vi "Proc_ccdIV.vi"(11 "error in (no error)":errorcluster, 12 "logfile":path, 13 "Database RefNum out":T1) -> (15 "error out":errorcluster)   [LabVIEW 2016]
uses:
  DBSHAND/private/vis/DatabaseHand_RefNum.ctl
  Common/public/vis/CMN_FVAR_action.ctl
  DBSHAND/private/vis/DatabaseHand_Element_Get(double).vi
  DBSHAND/private/vis/DatabaseHand_Element_Set(double).vi
  DBSHAND/private/vis/DatabaseHand_Element_Set(bool).vi
  DBSHAND/private/vis/DatabaseHand_Element_Get(I32).vi
  DBSHAND/private/vis/DatabaseHand_Element_Get(bool).vi
  DBSHAND/private/vis/DatabaseHand_Element_Set(I32).vi
panel:
  out "buf read":i32
  out "tot phys buffers":i32
  out "Total image Bytes":u32
  out "piece":i32
  out "virt bytes size":u32
  out "virt buf size":u32
  out "Total Pixels":u32
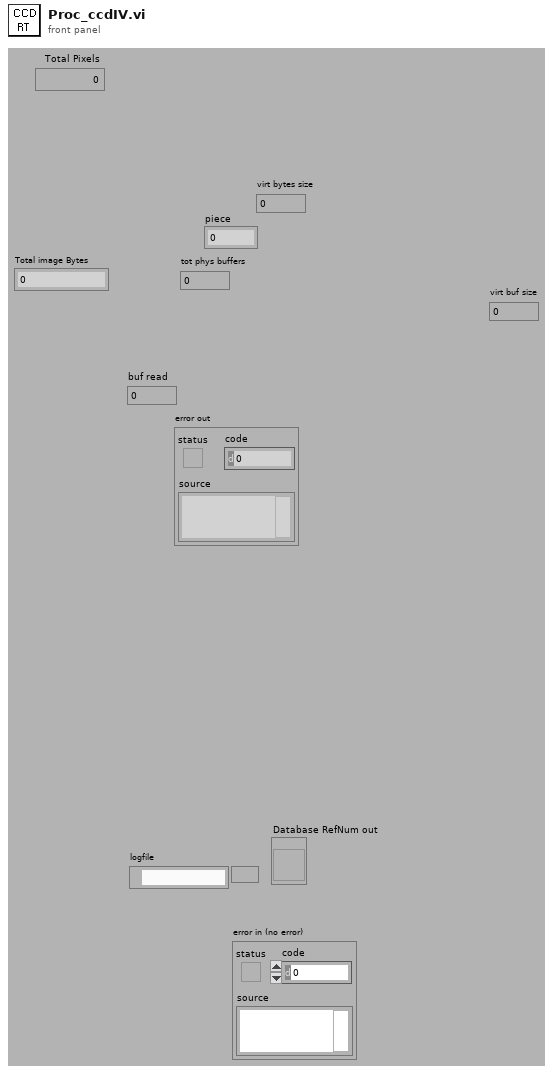
[diagram p1: front panel]
types:
  T1 = typedef "DatabaseHand_RefNum.ctl" = refnum<vi>
  T2 = typedef "CMN_FVAR_action.ctl" = enum16{"read", "write"}
  T3 = typedef "CMN_Buffers.ctl" = cluster{"TotalPixels":u32, "Total image bytes":u32, "Total Phys Buffers":u32, "virtual buf pixels":u32, "virtual bytes size":u32, "Remaining piece":u32, "Transfer_Buf_size":u32}
  T4 = cluster{"Name":string, "size (bytes)":u64, "pointer":u64, "Lock":bool}
  T5 = cluster{"pointer":u64, "size":u64, "progress":u32, "status":string}
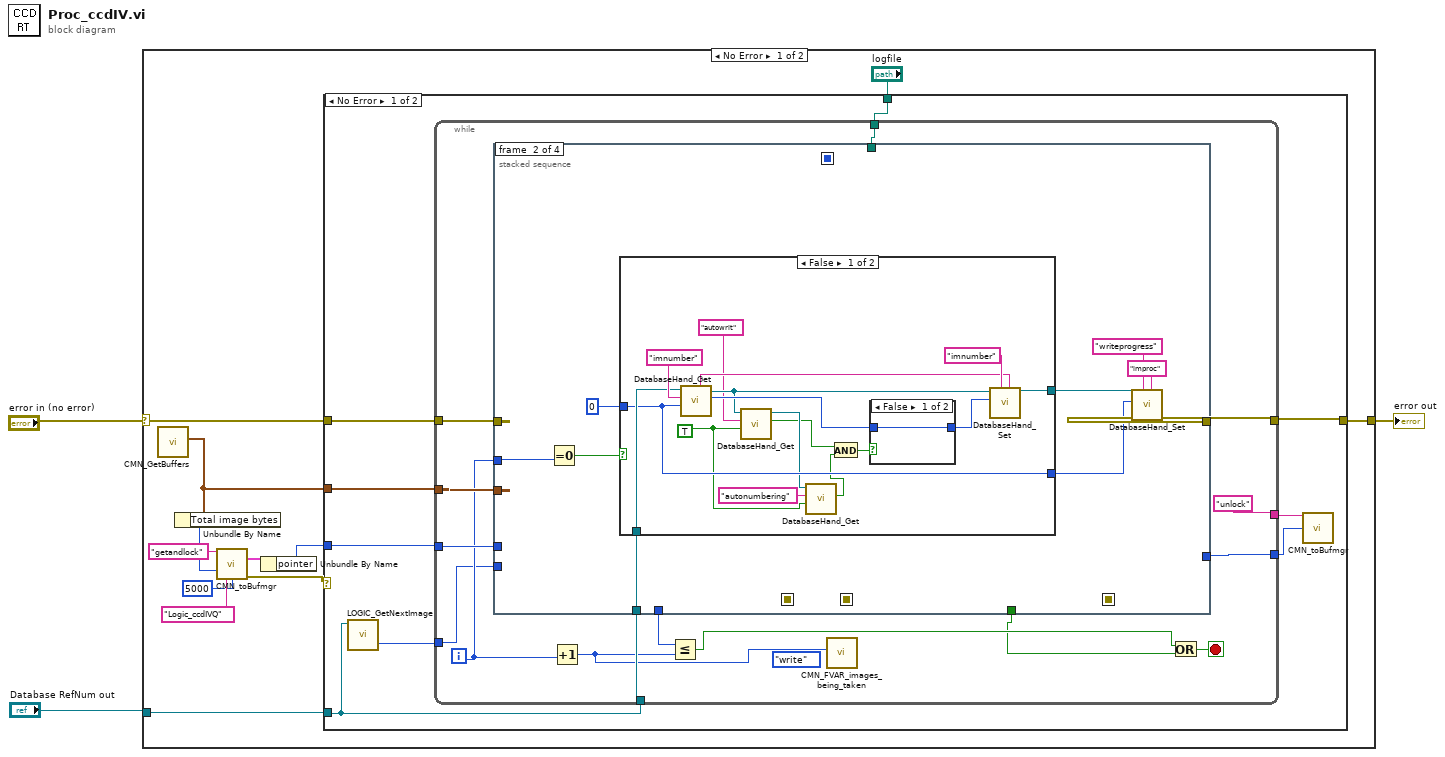
[diagram p0: block diagram]
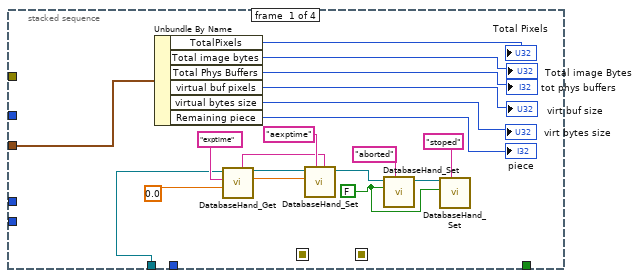
[diagram p2: hidden frame]
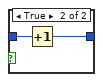
[diagram p3: hidden frame]
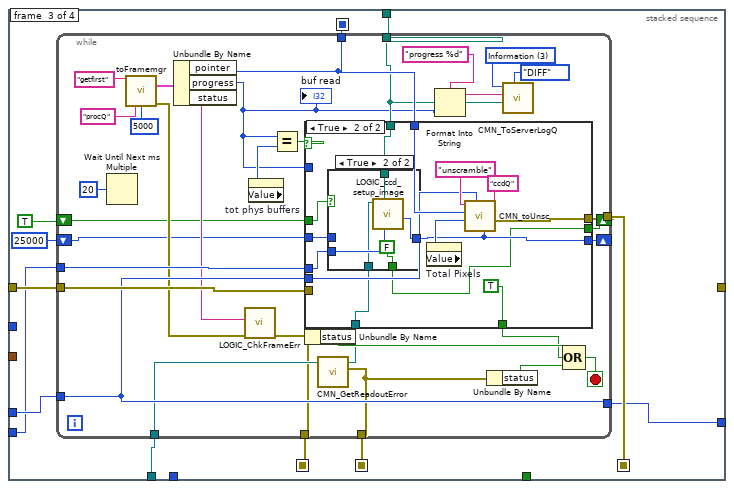
[diagram p5: hidden frame]
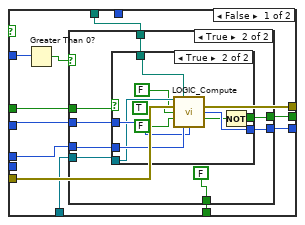
[diagram p6: hidden frame]
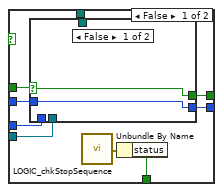
[diagram p7: hidden frame]
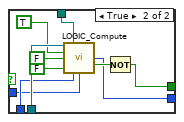
[diagram p8: hidden frame]
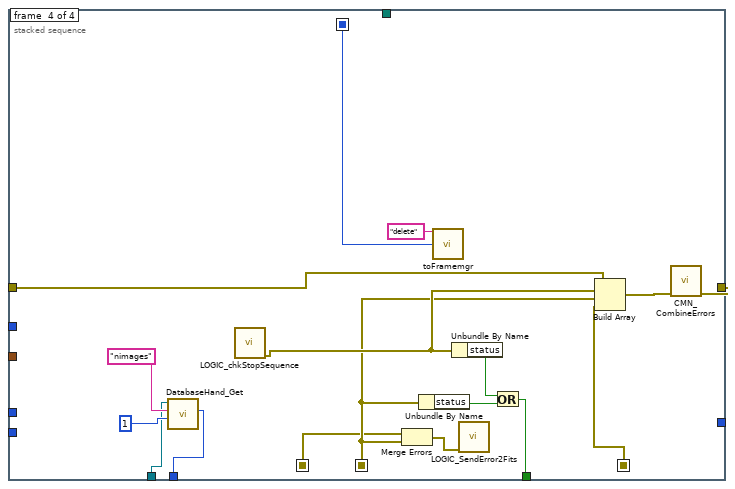
[diagram p11: hidden frame]
diagram:
  n1 = case shown="No Error" "error in (no error)" {
    selector: "error in (no error)" -> [w15 w223]
    tunnel: [w14 w223] -> w2
    tunnel: "Database RefNum out" -> [w4 _]
    frame No Error {
      n2 = call "CMN_GetBuffers.vi"() -> ("BuffersDimensions"=w5:T3)  [unwired: 2 in, 9 out]
      n3 = Unbundle By Name(w5) -> ("Total image bytes"=w12:u32)
      n4 = call "CMN_toBufmgr.vi"("command"="getandlock", "bufsize"=w12, "responseQ"="Logic_ccdIVQ", "ms timeout (-1)"=5000) -> ("buffer"=w10:T4, "error out"=w11:errorcluster)  [unwired: 4 in, 6 out]
      n5 = Unbundle By Name(w10) -> ("pointer"=w9:u64)
      n6 = case shown="No Error" w11 {
        selector: w11 -> [_ w222]
        tunnel: w15 -> [w24 _]
        tunnel: [w23 w222] -> w14
        tunnel: w5 -> [w22 _]
        tunnel: w9 -> [w21 _]
        tunnel: w4 -> [w17 _]
        tunnel: "logfile" -> [w18 _]
        frame No Error {
          n7 = call "LOGIC_GetNextImage.vi"("DBS Ref"=w17) -> ("raw bpp"=w16:i32)  [unwired: 10 out]
          n8 = while {
            tunnel: [w38] -> w23
            tunnel: w24 -> [w39]
            tunnel: w22 -> [w40]
            tunnel: w21 -> [w37]
            tunnel: [w36] -> w20
            tunnel: ["unlock" ("command")] -> w19
            tunnel: w17 -> [w34]
            tunnel: w18 -> [w33]
            tunnel: w16 -> [w29]
            i -> [w32]
            stop <- w27 stop-if-true
            n9 = stacked-sequence {
              seq-local: [_ _ w99 _] -> [_ _ _ w216]
              seq-local: [_ _ w98 _] -> [_ _ _ w217]
              seq-local: [_ _ w97 _] -> [_ _ _ w210]
              seq-local: [_ _ w96 _] -> [_ _ _ w211]
              tunnel: w40 -> [w42 _ _ _]
              tunnel: w39 -> [_ _ w100 w221]
              tunnel: [_ _ _ w219] -> w38
              tunnel: w37 -> [_ _ w95 _]
              tunnel: [_ _ w94 _] -> w36
              tunnel: w34 -> [w41 w62 w93 w206]
              tunnel: w33 -> [_ _ w92 _]
              tunnel: w32 -> [_ w63 _ _]
              tunnel: w29 -> [_ _ w91 _]
              tunnel: [_ _ _ w212] -> w26
              tunnel: [_ _ _ w205] -> w25
              frame #0 {
                w43 = FALSE
                n10 = Unbundle By Name(w42) -> ("TotalPixels"=→"Total Pixels":u32, "Total image bytes"=→"Total image Bytes":u32, "Total Phys Buffers"=→"tot phys buffers":u32, "virtual buf pixels"=→"virt buf size":u32, "virtual bytes size"=→"virt bytes size":u32, "Remaining piece"=→"piece":u32)
                n11 = call-poly "DatabaseHand_Get.vi"("default value"=0.0, "name"="exptime", "Database RefNum in"=w41) -> ("value"=w48:dbl, "Database RefNum out"=w53:T1, "group"=w50:string)  [unwired: 2 in, 4 out]
                n12 = call-poly "DatabaseHand_Set.vi"("group"=w50, "name"="aexptime", "value"=w48, "Database RefNum in"=w53) -> ("Database RefNum out"=w46:T1)  [unwired: 4 in, 3 out]
                n13 = call-poly "DatabaseHand_Set.vi"("name"="aborted", "value"=w43, "Database RefNum in"=w46) -> ("Database RefNum out"=w45:T1)  [unwired: 5 in, 3 out]
                n14 = call-poly "DatabaseHand_Set.vi"("name"="stoped", "value"=w43, "Database RefNum in"=w45) -> ()  [unwired: 5 in, 4 out]
              }
              frame #1 {
                n15 = Equal To 0?(x=w63) -> (x = 0?=w61:bool)
                n16 = case shown="False" w61 {
                  tunnel: [w78 w87] -> w67
                  tunnel: [w74 w88] -> w64
                  tunnel: w62 -> [w77 w87]
                  tunnel: 0 -> [w74 w88]
                  frame False {
                    w71 = TRUE
                    n17 = call-poly "DatabaseHand_Get.vi"("default value"=w74, "name"="imnumber", "Database RefNum in"=w77) -> ("value"=w81:i32, "Database RefNum out"=w76:T1, "group"=w82:string)  [unwired: 2 in, 4 out]
                    n18 = call-poly "DatabaseHand_Get.vi"("default value"=w71, "name"="autowrit", "Database RefNum in"=w76) -> ("value"=w69:bool, "Database RefNum out"=w72:T1)  [unwired: 2 in, 5 out]
                    n19 = call-poly "DatabaseHand_Get.vi"("default value"=w71, "name"="autonumbering", "Database RefNum in"=w72) -> ("value"=w70:bool)  [unwired: 2 in, 6 out]
                    n20 = And(x=w69, y=w70) -> (x .and. y?=w68:bool)
                    n21 = case shown="False" w68 {
                      tunnel: w81 -> [w84 w86]
                      tunnel: [w84 w85] -> w80
                      frame False {
                      }
                      frame True {
                        n22 = Increment(x=w86) -> (x+1=w85:i32)
                      }
                    }
                    n23 = call-poly "DatabaseHand_Set.vi"("group"=w82, "name"="imnumber", "value"=w80, "Database RefNum in"=w76) -> ("Database RefNum out"=w78:T1)  [unwired: 4 in, 3 out]
                  }
                  frame True {
                  }
                }
                n24 = call-poly "DatabaseHand_Set.vi"("group"="improc", "name"="writeprogress", "value"=w64, "Database RefNum in"=w67) -> ()  [unwired: 4 in, 4 out]
              }
              frame #2 {
                n25 = while {
                  tunnel: [w112] -> w97
                  tunnel: [w124] -> w98
                  tunnel: [w129] -> w99
                  tunnel: w100 -> [w130]
                  tunnel: [w120] -> w96
                  tunnel: w95 -> [w121]
                  tunnel: [w121] -> w94
                  tunnel: w93 -> [w116]
                  tunnel: w92 -> [w111]
                  tunnel: w91 -> [w115]
                  shift-right: [w102] -> _
                  shift-left: TRUE -> [w105]
                  shift-right: [w104] -> _
                  shift-left: 25000 ("usc_tmout") -> [w103]
                  stop <- w131 stop-if-true
                  w119 = u16 3 items=["command", "imediateReply", "Callback Reply", "Information"] ("type")
                  n26 = Wait Until Next ms Multiple(millisecond multiple=u32 20) -> ()  [unwired: 1 out]
                  n27 = call "toFramemgr.vi"("command"="getfirst", "responseQ"="procQ", "ms timeout (-1)"=5000) -> ("buffer"=w125:T5, "error out"=w114:errorcluster)  [unwired: 6 in, 5 out]
                  n28 = Unbundle By Name(w125) -> ("pointer"=w124:u64, "progress"=w106:u32, "status"=w113:string)
                  "buf read" <- w106
                  n29 = call "LOGIC_ChkFrameErr.vi"("error in"=w114, "frame status"=w113) -> ("error out"=w112:errorcluster)  [unwired: 9 out]
                  n30 = property on="tot phys buffers" class="DigNum (strict)"() -> ("Value"=w107:i32)  [unwired: 2 in, 2 out]
                  n31 = Equal?(x=w106, y=w107) -> (x = y?=w122:bool)
                  n32 = case shown="True" w122 {
                    tunnel: w130 -> [w142 _]
                    tunnel: [w142 w194] -> w129
                    tunnel: w124 -> [_ w195]
                    tunnel: w121 -> [_ w192]
                    tunnel: w116 -> [w137 w188]
                    tunnel: w111 -> [w136 w190]
                    tunnel: w115 -> [w135 w189]
                    tunnel: [w141 TRUE] -> w110
                    tunnel: w106 -> [w140 _]
                    tunnel: w105 -> [w139 w185]
                    tunnel: [w138 w184] -> w102
                    tunnel: [w134 w186] -> w104
                    tunnel: w103 -> [w133 w187]
                    frame False {
                      (unwired) FALSE
                      n33 = Greater Than 0?(x=w140) -> (x > 0?=w132:bool)
                      n34 = case shown="True" w132 {
                        tunnel: [w150 FALSE ("status")] -> w141
                        tunnel: w139 -> [w143 w165]
                        tunnel: [w147 w169] -> w138
                        tunnel: w137 -> [w149 w171]
                        tunnel: w136 -> [w148 w168]
                        tunnel: w135 -> [w146 w167]
                        tunnel: [w145 w166] -> w134
                        tunnel: w133 -> [w144 w164]
                        frame False {
                          n35 = case shown="False" w143 {
                            selector: w143 -> [w152 _]
                            tunnel: w149 -> [_ w163]
                            tunnel: w148 -> [_ w162]
                            tunnel: [w152 w157] -> w147
                            tunnel: w146 -> [_ w156]
                            tunnel: [w153 w155] -> w145
                            tunnel: w144 -> [w153 w154]
                            frame False {
                            }
                            frame True {
                              n36 = call "LOGIC_Compute.vi"("Database RefNum in"=w163, "log_file"=w162, "expstart"=TRUE, "readstart"=FALSE, "readend"=FALSE, "raw bpp"=w156, "usc_tmout in"=w154) -> ("usc_tmout"=w155:i32, "created"=w158:bool)  [unwired: 1 in, 6 out]
                              n37 = Not(x=w158) -> (.not. x?=w157:bool)
                            }
                          }
                          n38 = call "LOGIC_chkStopSequence.vi"() -> ("error out"=w151:errorcluster)  [unwired: 11 out]
                          n39 = Unbundle By Name(w151) -> ("status"=w150:bool)
                        }
                        frame True {
                          n40 = case shown="True" w165 {
                            selector: w165 -> [w173 _]
                            tunnel: w171 -> [_ w177]
                            tunnel: [w173 w178] -> w169
                            tunnel: w168 -> [_ w183]
                            tunnel: w167 -> [_ w182]
                            tunnel: [w172 w180] -> w166
                            tunnel: w164 -> [w172 w181]
                            frame False {
                            }
                            frame True {
                              n41 = call "LOGIC_Compute.vi"("Database RefNum in"=w177, "log_file"=w183, "expstart"=FALSE, "readstart"=TRUE, "readend"=FALSE, "raw bpp"=w182, "usc_tmout in"=w181) -> ("usc_tmout"=w180:i32, "created"=w179:bool)  [unwired: 1 in, 6 out]
                              n42 = Not(x=w179) -> (.not. x?=w178:bool)
                            }
                          }
                        }
                      }
                    }
                    frame True {
                      n43 = case shown="True" w185 {
                        selector: w185 -> [w198 _]
                        tunnel: w190 -> [_ w204]
                        tunnel: w189 -> [_ w203]
                        tunnel: w188 -> [_ w202]
                        tunnel: w187 -> [w199 _]
                        tunnel: [w199 w201] -> w186
                        tunnel: [w198 FALSE] -> w184
                        frame False {
                        }
                        frame True {
                          n44 = call "LOGIC_ccd_setup_image.vi"("raw bpp"=w203, "log_file"=w204, "Database RefNum in"=w202) -> ("usc_tmout"=w201:i32)  [unwired: 1 in, 7 out]
                        }
                      }
                      n45 = property on="Total Pixels" class="DigNum (strict)"() -> ("Value"=w193:u32)  [unwired: 2 in, 2 out]
                      n46 = call "CMN_toUnsc.vi"("responseQ"="ccdQ", "ms timeout (-1)"=w186, "location 2"=w192, "ele Read"=w193, "location"=w195, "command"="unscramble") -> ("response"=w194:errorcluster)  [unwired: 3 in, 2 out]
                    }
                  }
                  n47 = Unbundle By Name(w112) -> ("status"=w123:bool)
                  n48 = call "CMN_GetReadoutError.vi"("Database RefNum in"=w116) -> ("readout_error"=w120:errorcluster)  [unwired: 1 in, 9 out]
                  n49 = Format Into String(format string="progress %d", w106) -> (resulting string=w117:string)  [unwired: 2 in, 1 out]
                  n50 = Unbundle By Name(w120) -> ("status"=w108:bool)
                  n51 = call "CMN_ToServerLogQ.vi"("Mode"=enum16{"ALL", "DIFF"}."DIFF", "file"=w111, "string"=w117, "type"=w119) -> ()  [unwired: 2 in, 5 out]
                  n52 = Compound Arithmetic op=OR(w123, w110, w108) -> (w131:bool)
                }
              }
              frame #3 {
                n53 = call-poly "DatabaseHand_Get.vi"("default value"=1 ("ImageNumber"), "name"="nimages", "Database RefNum in"=w206) -> ("value"=w205:i32)  [unwired: 2 in, 6 out]
                n54 = call "LOGIC_chkStopSequence.vi"() -> ("error out"=w215:errorcluster)  [unwired: 11 out]
                n55 = Merge Errors(w210, w211) -> (w209:errorcluster)
                n56 = Unbundle By Name(w211) -> ("status"=w213:bool)
                n57 = call "toFramemgr.vi"("command"="delete", "bufpointer"=w217) -> ()  [unwired: 7 in, 7 out]
                n58 = Unbundle By Name(w215) -> ("status"=w214:bool)
                n59 = call "LOGIC_SendError2Fits.vi"("error in (no error)"=w209) -> ()  [unwired: 11 out]
                n60 = Or(x=w214, y=w213) -> (x .or. y?=w212:bool)
                n61 = Build Array(w221, w215, w211, w216) -> (w220:errorcluster[])
                n62 = call "CMN_CombineErrors.vi"("Errors"=w220) -> ("error out"=w219:errorcluster)  [unwired: 10 out]
              }
            }
            n63 = Increment(x=w32) -> (x+1=w31:i32)
            n64 = Less Or Equal?(x=w25, y=w31) -> (x <= y?=w28:bool)
            n65 = call "CMN_FVAR_images_being_taken.vi"("value in"=w31, "action"=CMN_FVAR_action."write") -> ()  [unwired: 9 out]
            n66 = Or(x=w28, y=w26) -> (x .or. y?=w27:bool)
          }
          n67 = call "CMN_toBufmgr.vi"("command"=w19, "bufpointer"=w20) -> ()  [unwired: 6 in, 8 out]
        }
        frame Error {
        }
      }
    }
    frame Error {
    }
  }
  "error out" <- w2
